vi "Save-Recall Instrument Settings.vi"(8 "error in (no error)":errorcluster, 9 "Save Number (0)":u16(ring) items=["0", "1", "2", "3", "4", "5", "6", "7", "8", "9", "10"], 10 "Recall or Save (0:Recall)":u16(ring) items=["Recall", "Save"], 11 "VISA resource name":refnum<visa-resource-name>) -> (0 "error out":errorcluster, 3 "VISA resource name out":refnum<visa-resource-name>)   [LabVIEW 2013, in "Stanford Research CG635.lvlib"]
doc: "Recalls or Saves Instrument settings depending on parameter <B>Recall or Save</B>. Recalls or saves from or to the save file <B>Save Number</B>, respectively."
uses:
  <instrlib>/Stanford Research CG635/Stanford Research CG635.lvlib
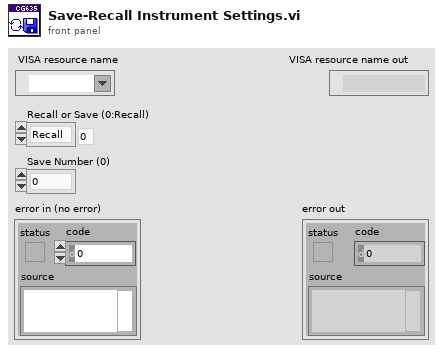
[diagram p1: front panel]
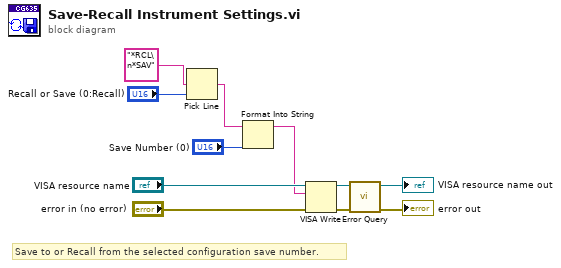
[diagram p0: block diagram]
diagram:
  # "Save to or Recall from the selected configuration save number."
  n1 = Pick Line(multi-line string="*RCL\n*SAV", line index="Recall or Save (0:Recall)") -> (output string=w6:string)  [unwired: 1 in]
  n2 = Format Into String(initial string=w6, "Save Number (0)") -> (resulting string=w8:string)  [unwired: 2 in, 1 out]
  n3 = VISA Write(VISA resource name="VISA resource name", write buffer=w8, error in (no error)="error in (no error)") -> (VISA resource name out=w4:refnum<visa-resource-name>, error out=w3:errorcluster)  [unwired: 1 out]
  n4 = call <instrlib>:"Error Query.vi"("error in (no error)"=w3, "VISA resource name"=w4) -> ("error out"=→"error out":errorcluster, "VISA resource name out"=→"VISA resource name out":refnum<visa-resource-name>)  [unwired: 6 in, 2 out]
